vi "SelectElementToWrite.vi"(8 "error in (no error)":errorcluster, 11 "ArrayElementScripter in":refnum<class "ArrayElementScripter.lvclass">) -> (0 "error out":errorcluster, 3 "ArrayElementScripter out":refnum<class "ArrayElementScripter.lvclass">)   [LabVIEW 2021, in "MemberVICreation.lvlib" / "ArrayElementScripter.lvclass"]
uses:
  <resource>/Framework/Providers/LVClassLibrary/NewAccessors/ArrayElementScripter/ArrayElementScripter.lvclass
  <resource>/Framework/Providers/LVClassLibrary/NewAccessors/BaseAccessorScripter/BaseAccessorScripter.lvclass
  <resource>/Framework/Providers/LVClassLibrary/NewAccessors/MemberVICreation.lvlib
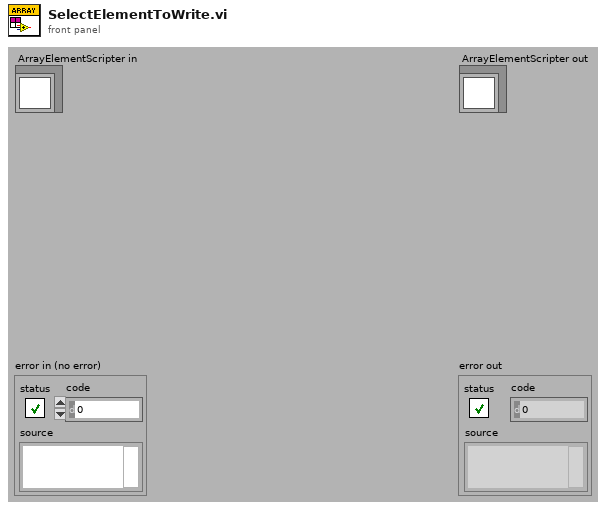
[diagram p1: front panel]
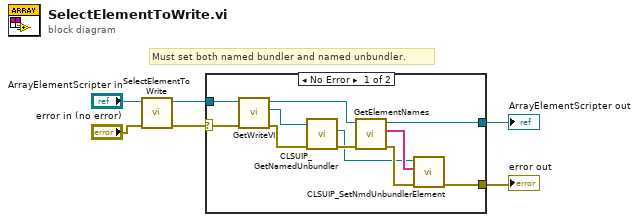
[diagram p0: block diagram]
diagram:
  # "Must set both named bundler and named unbundler."
  n1 = call-parent "SelectElementToWrite.vi"("error in (no error)"="error in (no error)", "BaseAccessorScripter in"="ArrayElementScripter in") -> ("error out"=w4:errorcluster, "BaseAccessorScripter out"=w2:refnum<class "ArrayElementScripter.lvclass">)  [unwired: 8 out]
  n2 = case shown="No Error" w4 {
    selector: w4 -> [w9 w19]
    tunnel: [w12 w19] -> w1
    tunnel: [w17 w18] -> w3
    tunnel: w2 -> [w10 w18]
    frame No Error {
      n3 = call-dynamic "GetWriteVI.vi"("error in (no error)"=w9, "BaseAccessorScripter in"=w10) -> ("error out"=w8:errorcluster, "Write VI"=w7:refnum<vi>, "BaseAccessorScripter out"=w11:refnum<class "ArrayElementScripter.lvclass">)  [unwired: 7 out]
      n4 = call <resource>:"CLSUIP_GetNamedUnbundler.vi"("error in (no error)"=w8, "VI Refnum"=w7) -> ("error out"=w16:errorcluster, "NmdBundler Ref"=w13:refnum<vi>)  [unwired: 8 out]
      n5 = call-dynamic "GetElementNames.vi"("error in (no error)"=w16, "ArrayElementScripter in"=w11) -> ("error out"=w15:errorcluster, "Element Names"=w14:string[], "ArrayElementScripter out"=w17:refnum<class "ArrayElementScripter.lvclass">)  [unwired: 7 out]
      n6 = call <resource>:"CLSUIP_SetNmdUnbundlerElement.vi"("error in (no error)"=w15, "Element Names"=w14, "NmdUnbundler Ref"=w13) -> ("error out"=w12:errorcluster)  [unwired: 8 out]
    }
    frame Error {
    }
  }
  "error out" <- w1
  "ArrayElementScripter out" <- w3
